vi "BulletFrame.vi"(2 "error in":errorcluster caption="错误输入（无错误）", 3 "StrIn":string="2D后视视图") -> (0 "error out":errorcluster caption="错误输出", 1 "结果":bool)   [LabVIEW 2013]
panel:
  in  "Fail":bool
  in  "Pass":bool
  out "CurrentView":string
  # "请看LVDS显示屏，与黑色框中视图是否一致"
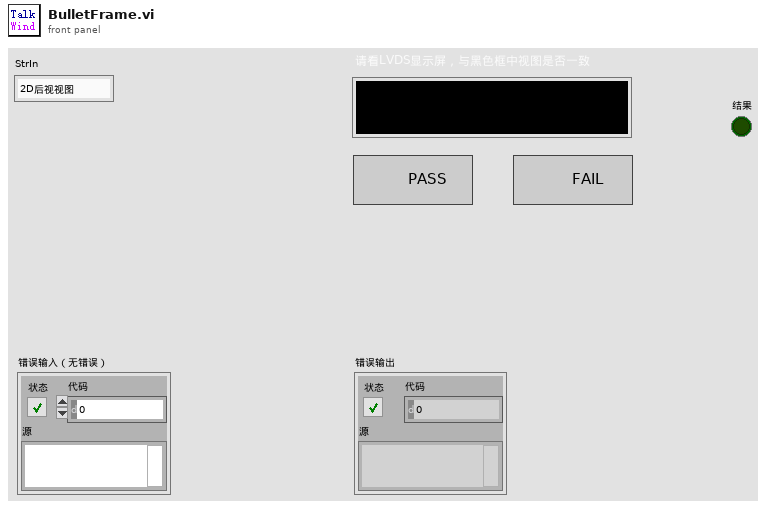
[diagram p1: front panel]
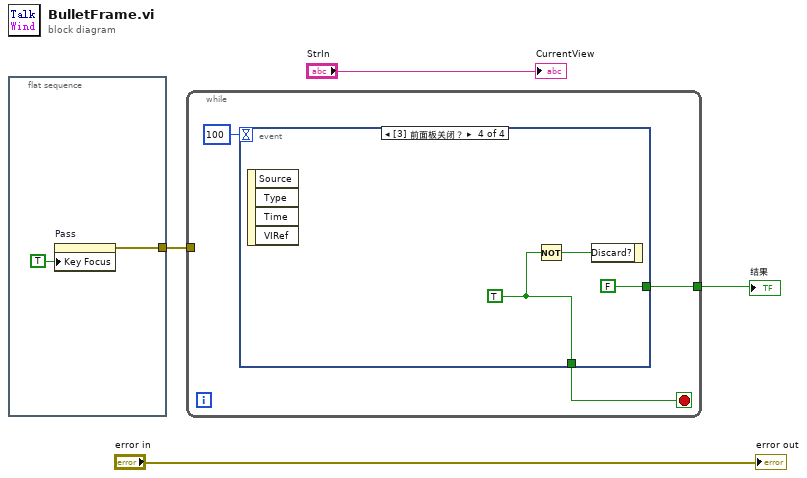
[diagram p0: block diagram]
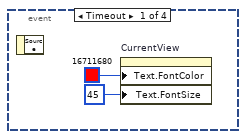
[diagram p2: hidden frame]
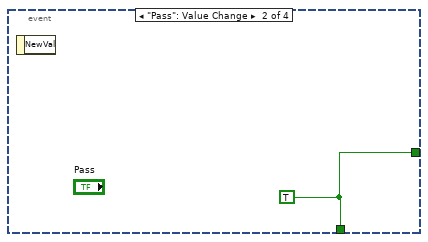
[diagram p3: hidden frame]
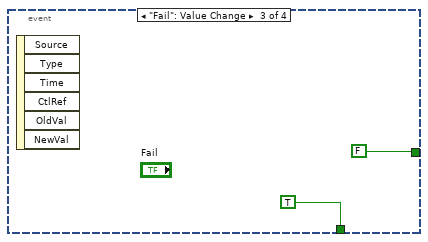
[diagram p4: hidden frame]
diagram:
  n1 = flat-sequence {
    tunnel: [w5] -> w1
    frame #0 {
      n2 = property on="Pass" class="Bool"("Key Focus"=TRUE ("键选中")) -> (error out=w5:errorcluster)  [unwired: 2 in, 1 out]
    }
  }
  n3 = while {
    tunnel: [w8] -> w3
    tunnel: w1 -> [_]
    stop <- w9 stop-if-true
    n4 = event shown="[3] 前面板关闭？" {
      selector: _ -> [_ _ _ _]
      dyn-events: _ -> [_ _ _ _]
      timeout: 100 -> [_ _ _ _]
      tunnel: [_ w12 TRUE w16] -> w9
      tunnel: [_ w12 FALSE FALSE] -> w8
      event Timeout {
        n5 = event-data() -> ()  [unwired: 1 in, 1 out]
        n6 = property on="CurrentView" class="Str"("Text.FontColor"=u32 16711680, "Text.FontSize"=u32 45 ("文本.字体:字号")) -> ()  [unwired: 2 in, 2 out]
      }
      event "Pass": Value Change {
        w12 = TRUE
        n7 = event-data() -> ()  [unwired: 1 in, 1 out]
      }
      event "Fail": Value Change {
        n8 = event-data() -> ()  [unwired: 1 in, 6 out]
      }
      event Panel Close? {
        w16 = TRUE
        n9 = event-data() -> ()  [unwired: 1 in, 4 out]
        n10 = Not(x=w16) -> (.not. x?=w15:bool)
        n11 = event-data("Discard?"=w15) -> ()  [unwired: 1 in, 1 out]
      }
    }
  }
  "结果" <- w3
  "CurrentView" <- "StrIn"
  "error out" <- "error in"
